vi "State Select.vi"(8 "State In":string, 9 "error in (no error)":errorcluster, 11 "States Array In":string[](array[string])) -> (0 "State Out":string, 3 "States Array Out":string[](array[string]))   [LabVIEW 2020]
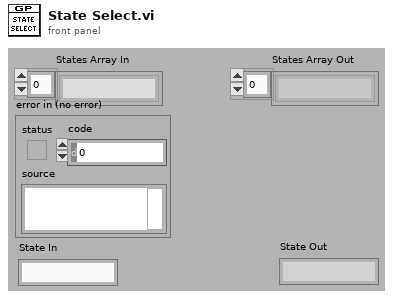
[diagram p1: front panel]
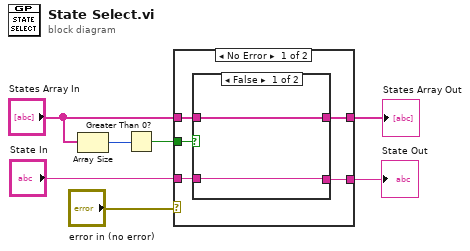
[diagram p0: block diagram]
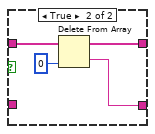
[diagram p2: hidden frame]
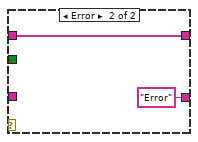
[diagram p3: hidden frame]
diagram:
  n1 = Array Size(array="States Array In") -> (size(s)=w7:i32)
  n2 = Greater Than 0?(x=w7) -> (x > 0?=w6:bool)
  n3 = case shown="No Error" "error in (no error)" {
    tunnel: w6 -> [w12 _]
    tunnel: "States Array In" -> [w11 w19]
    tunnel: "State In" -> [w10 _]
    tunnel: [w9 "Error" ("String")] -> w3
    tunnel: [w8 w19] -> w2
    frame No Error {
      n4 = case shown="False" w12 {
        tunnel: w11 -> [w14 w18]
        tunnel: w10 -> [w13 _]
        tunnel: [w13 w17] -> w9
        tunnel: [w14 w16] -> w8
        frame False {
        }
        frame True {
          n5 = Delete From Array(array=w18, index=0) -> (deleted portion=w17:string, array with subset deleted=w16:string[])  [unwired: 1 in]
        }
      }
    }
    frame Error {
    }
  }
  "State Out" <- w3
  "States Array Out" <- w2
